vi "readwrite.vi"(8 "error in (no error)":errorcluster, 9 "Command ID":i32, 10 "Command":string, 11 "Serial port":refnum<visa-resource-name>) -> (0 "error out":errorcluster, 1 "success":bool, 2 "responses":string[](array[string]), 3 "Serial port out":refnum<visa-resource-name>)   [LabVIEW 2012]
panel:
  out "concatenated string":string
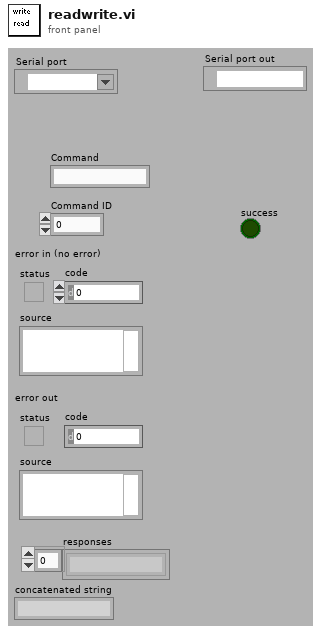
[diagram p1: front panel]
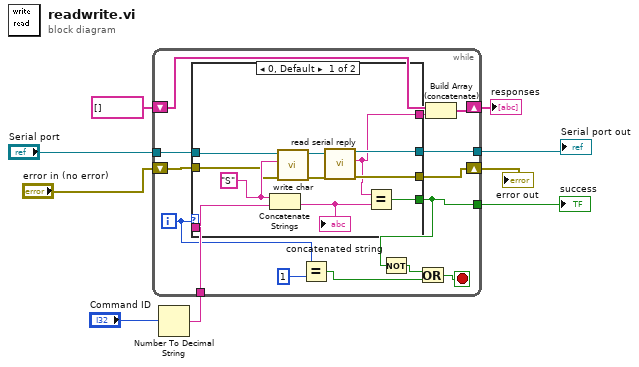
[diagram p0: block diagram]
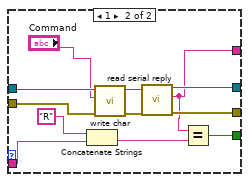
[diagram p2: hidden frame]
diagram:
  n1 = Number To Decimal String(number="Command ID") -> (decimal integer string=w5:string)  [unwired: 1 in]
  n2 = while {
    tunnel: "Serial port" -> [w23]
    tunnel: [w22] -> w8
    tunnel: [w15] -> w7
    tunnel: w5 -> [w21]
    shift-right: [w13] -> w3
    shift-left: "error in (no error)" -> [w14]
    shift-right: [w12] -> w1
    shift-left: string[] [] -> [w10]
    i -> [w20]
    stop <- w17 stop-if-true
    n3 = case shown="0, Default" w20 {
      tunnel: w23 -> [w32 w44]
      tunnel: [w31 w43] -> w22
      tunnel: [w30 w42] -> w15
      tunnel: w21 -> [w29 w41]
      tunnel: w14 -> [w26 w38]
      tunnel: [w25 w37] -> w13
      tunnel: [w24 w36] -> w11
      frame 0, Default {
        w28 = "S"
        n4 = Concatenate Strings(w28, w29) -> (w27:string)
        "concatenated string" <- w27
        n5 = call "write char.vi"("error in (no error)"=w26, "write buffer"=w28, "Serial port"=w32) -> ("error out"=w34:errorcluster, "Serial Port"=w33:refnum<visa-resource-name>)  [unwired: 6 in, 1 out]
        n6 = call "read serial reply.vi"("error in (no error)"=w34, "Serial Port"=w33) -> ("error out"=w25:errorcluster, "reply"=w24:string, "Serial Port out"=w31:refnum<visa-resource-name>)  [unwired: 7 in]
        n7 = Equal?(x=w24, y=w27) -> (x = y?=w30:bool)
      }
      frame 1 {
        n8 = Concatenate Strings("R", w41) -> (w40:string)
        n9 = call "write char.vi"("error in (no error)"=w38, "write buffer"="Command", "Serial port"=w44) -> ("error out"=w46:errorcluster, "Serial Port"=w45:refnum<visa-resource-name>)  [unwired: 6 in, 1 out]
        n10 = call "read serial reply.vi"("error in (no error)"=w46, "Serial Port"=w45) -> ("error out"=w37:errorcluster, "reply"=w36:string, "Serial Port out"=w43:refnum<visa-resource-name>)  [unwired: 7 in]
        n11 = Equal?(x=w36, y=w40) -> (x = y?=w42:bool)
      }
    }
    n12 = Equal?(x=w20, y=1) -> (x = y?=w18:bool)
    n13 = Not(x=w15) -> (.not. x?=w16:bool)
    n14 = Or(x=w16, y=w18) -> (x .or. y?=w17:bool)
    n15 = Build Array (concatenate)(w10, w11) -> (w12:string[])
  }
  "Serial port out" <- w8
  "success" <- w7
  "error out" <- w3
  "responses" <- w1
